vi "Create New Switch.vi"(0 "VISA resource name":refnum<visa-resource-name>, 1 "Address (\"1\")":string="\"1\"", 2 "Order (0)":i32, 5 "Name (\"NewSwitch\")":string="\"NewSwitcher\"", 7 "Switch Type (0: stBNCOutput)":i32(ring) items=["stBNCOutput", "stBNCInput", "stXLROutput", "stXLRInput"], 9 "Control Type (0: ctSerial)":i32(ring) items=["ctSerial", "ctTCPIP"], 11 "error in (no error)":errorcluster, 12 "ChainID (0)":i32) -> (4 "VISA resource name out":refnum<visa-resource-name>, 15 "error out":errorcluster)   [LabVIEW 2014, in "Stanford Research SR1.lvlib"]
doc: "Adds a new switch with the specified name and options to the switcher network."
uses:
  Stanford Research SR1.lvlib
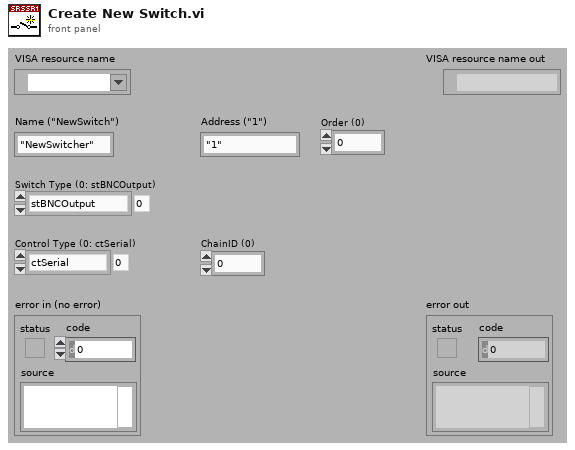
[diagram p1: front panel]
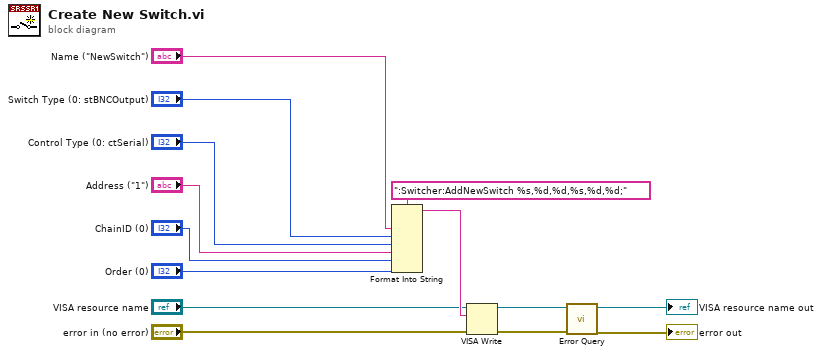
[diagram p0: block diagram]
diagram:
  n1 = Format Into String(format string=":Switcher:AddNewSwitch %s,%d,%d,%s,%d,%d;", "Name (\"NewSwitch\")", "Switch Type (0: stBNCOutput)", "Control Type (0: ctSerial)", "Address (\"1\")", "ChainID (0)", "Order (0)") -> (resulting string=w10:string)  [unwired: 2 in, 1 out]
  n2 = VISA Write(VISA resource name="VISA resource name", write buffer=w10, error in (no error)="error in (no error)") -> (VISA resource name out=w7:refnum<visa-resource-name>, error out=w6:errorcluster)  [unwired: 1 out]
  n3 = call "Error Query.vi"("error in (no error)"=w6, "VISA resource name"=w7) -> ("error out"=→"error out":errorcluster, "VISA resource name out"=→"VISA resource name out":refnum<visa-resource-name>)  [unwired: 6 in, 2 out]
